vi "Write Ideal Values .vi"(8 "Error In":errorcluster, 10 "Ideal Values":T1, 11 "INL DNL Test in":refnum<class "INL DNL Test.lvclass">) -> (0 "Error Out":errorcluster, 3 "INL DNL Test out":refnum<class "INL DNL Test.lvclass">)   [LabVIEW 2020, in "INL DNL Test.lvclass"]
uses:
  INL DNL Test.lvclass
  Device/Parent/Typedef/Data Cluster.ctl
  INL DNL Test.lvclass/INL DNL Test.ctl
  Device/Parent/Device.lvclass
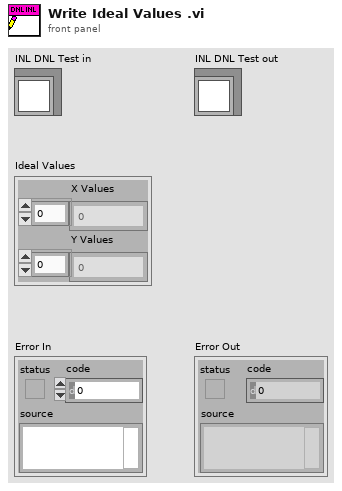
[diagram p1: front panel]
types:
  T1 = typedef "Device.lvclass/Data Cluster.ctl" = cluster{"X Values":dbl[], "Y Values":dbl[]}
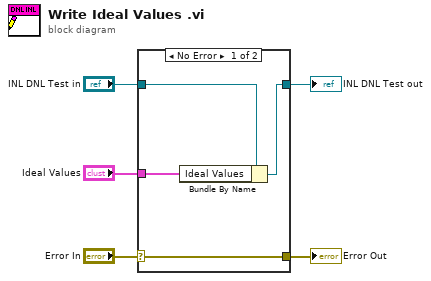
[diagram p0: block diagram]
diagram:
  n1 = case shown="No Error" "Error In" {
    selector: "Error In" -> [w9 w10]
    tunnel: [w9 w10] -> w4
    tunnel: [w7 w11] -> w2
    tunnel: "INL DNL Test in" -> [w8 w11]
    tunnel: "Ideal Values" -> [w6 _]
    frame No Error {
      n2 = Bundle By Name(cluster=w8, "Ideal Values"=w6) -> (w7:refnum<class "INL DNL Test.lvclass">)
    }
    frame Error {
    }
  }
  "Error Out" <- w4
  "INL DNL Test out" <- w2
